vi "DriveLimit-Control.vi"(1 "Limit":dbl=0.75, 2 "Scale Limit":dbl=0.5, 3 "Enable Limit":bool=TRUE, 4 "Controler Value Input":dbl) -> (0 "OUTPUT VALUE":dbl)   [LabVIEW 2015]
panel:
  # "This limit is used affter it is timed by Scale Limit"
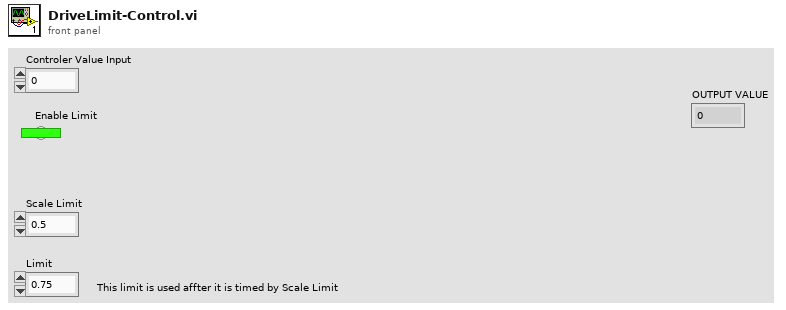
[diagram p1: front panel]
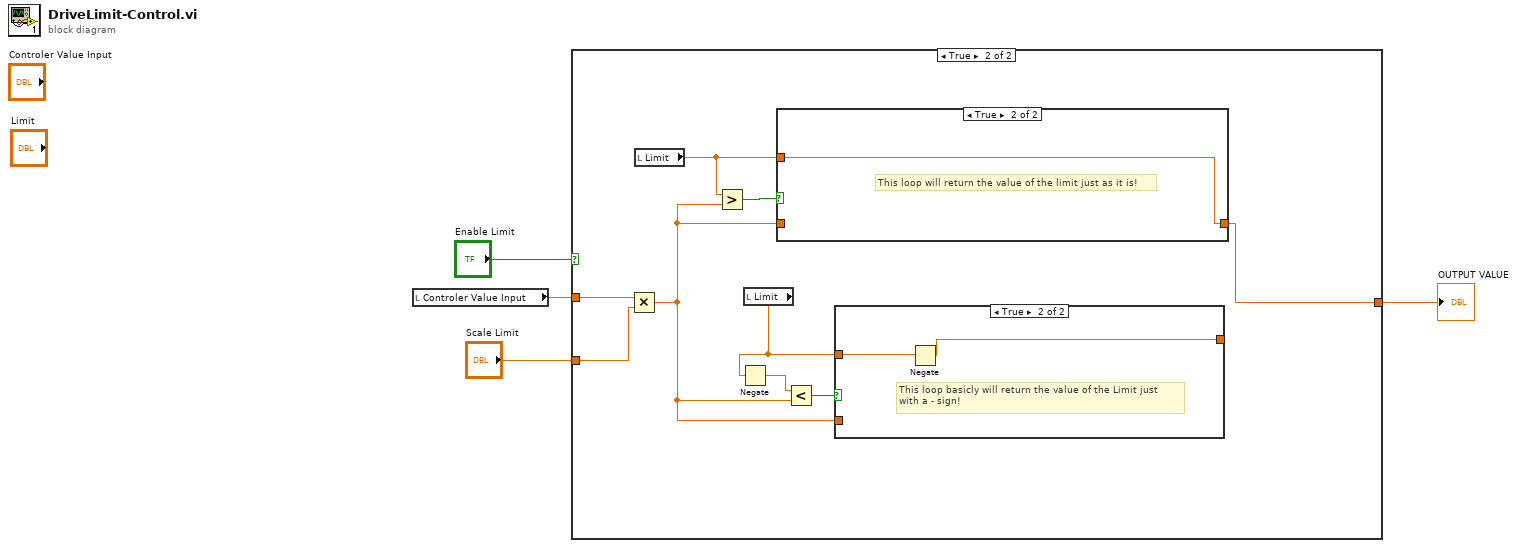
[diagram p0: block diagram]
diagram:
  n1 = local read "Controler Value Input"() -> (w3:dbl)
  n2 = case shown="True" "Enable Limit" {
    tunnel: w3 -> [w5 w14]
    tunnel: [w5 w11] -> w2
    tunnel: "Scale Limit" -> [_ w6]
    frame False {
    }
    frame True {
      n3 = Multiply(x=w14, y=w6) -> (x*y=w9:dbl)
      n4 = local read "Limit"() -> (w13:dbl)
      n5 = Greater?(x=w13, y=w9) -> (0:w12:bool)
      n6 = local read "Limit"() -> (w7:dbl)
      n7 = Negate(x=w7) -> (-x=w8:dbl)
      n8 = case shown="True" w12 {
        tunnel: w9 -> [w18 _]
        tunnel: [w18 w19] -> w11
        tunnel: w13 -> [_ w19]
        frame False {
        }
        frame True {
          # "This loop will return the value of the limit just as it is!"
        }
      }
      n9 = Less?(x=w8, y=w9) -> (x < y?=w10:bool)
      n10 = case shown="True" w10 {
        tunnel: w9 -> [w15 _]
        tunnel: [w15 w16] -> _
        tunnel: w7 -> [_ w17]
        frame False {
        }
        frame True {
          # "This loop basicly will return the value of the Limit just \nwith a - sign!"
          n11 = Negate(x=w17) -> (-x=w16:dbl)
        }
      }
    }
  }
  "OUTPUT VALUE" <- w2
